vi "Open Library if Not in Memory.vi"(8 "error in (no error)":errorcluster, 11 "Path":path) -> (0 "error out":errorcluster, 3 "Library Ref":refnum<vi>, 5 "Opened?":bool)   [LabVIEW 2020, in "VI Properties Editor.lvlib"]
doc: "Opens the library specified by <B>Path</B> only if it was not already in memory."
uses:
  VI Properties Editor.lvlib
  <vilib>/AdvancedString/Delimited String to 1D String Array (string).vi
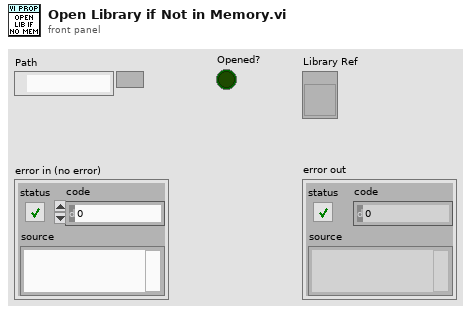
[diagram p1: front panel]
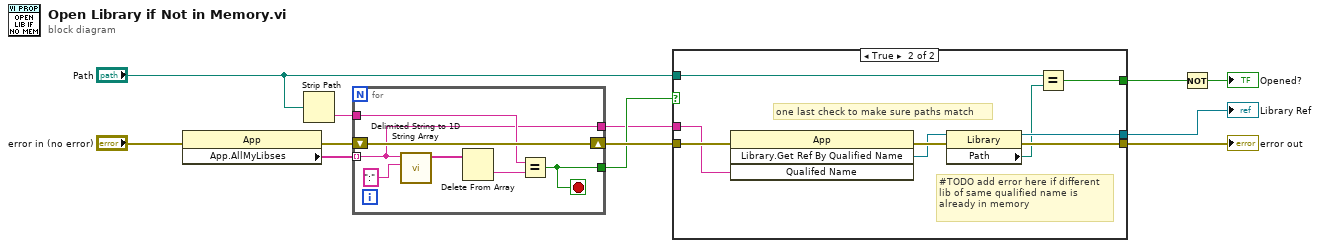
[diagram p0: block diagram]
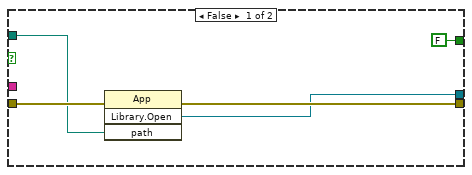
[diagram p2: hidden frame]
diagram:
  n1 = property class="App"(error in="error in (no error)") -> (error out=w12:errorcluster, "App.AllMyLibses"=w10:string[])  [unwired: 1 in, 1 out]
  n2 = Strip Path(path="Path") -> (name=w4:string)  [unwired: 1 out]
  n3 = for {
    tunnel: w10 -> [w13] mode=indexing
    tunnel: [w18] -> w3
    shift-right: [w19] -> w11
    shift-left: w12 -> [w19]
    tunnel: w4 -> [w17]
    tunnel: [w13] -> w2
    stop <- w18 stop-if-true
    n4 = call-poly <vilib>:"Delimited String to 1D String Array.vi"("delimiter"=":", "delimited string"=w13) -> ("string array"=w15:string[])  [unwired: 9 in]
    n5 = Delete From Array(array=w15) -> (deleted portion=w14:string)  [unwired: 2 in, 1 out]
    n6 = Equal?(x=w17, y=w14) -> (x = y?=w18:bool)
  }
  n7 = case shown="True" w3 {
    tunnel: w11 -> [w24 w33]
    tunnel: [w23 w29] -> w9
    tunnel: [w22 w26] -> w8
    tunnel: "Path" -> [w21 w28]
    tunnel: w2 -> [_ w32]
    tunnel: [FALSE w27] -> w1
    frame False {
      n8 = invoke class="App" method="Library.Open"(error in=w24, "path"=w21) -> (error out=w23:errorcluster, "Open Library"=w22:refnum<vi>)  [unwired: 2 in, 2 out]
    }
    frame True {
      # "one last check to make sure paths match"
      # "#TODO add error here if different lib of same qualified name is already in memory"
      n9 = invoke class="App" method="Library.Get Ref By Qualified Name"(error in=w33, "Qualifed Name"=w32) -> (error out=w31:errorcluster, "Library.Get Ref By Qualified Name"=w30:refnum<vi>)  [unwired: 2 in, 2 out]
      n10 = property class="Library"(reference=w30, error in=w31) -> (reference out=w26:refnum<vi>, error out=w29:errorcluster, "Path"=w25:path)
      n11 = Equal?(x=w28, y=w25) -> (x = y?=w27:bool)
    }
  }
  "error out" <- w9
  "Library Ref" <- w8
  n12 = Not(x=w1) -> (.not. x?=→"Opened?":bool)
